vi "ModifyCamGainOnFly.vi"() -> (11 "Waveform Graph":T1(graph)={"Starting Value"=0.0, "Incremental Value"=1.0, "Histogram"=[36, 1982, 49222, 315462, 721902, 687030, 535519, 277999, 136964, 72699, 42936, 24297, 19870, 14020, 10724, 8169, 7364, 6885, 8983, 9078, 8040, 5942, 4163, 2700, 2224, 1518, 1184, 962, 794, 840, 791, 692, 704, 627, 576, 578, 599, 535, 562, 517, 433, 498, 495, 523, 508, 500, 424, 516, 521, 534, 536, 550, 473, 579, 637, 766, 994, 1390, 2263, 3532, 4826, 6338, 7904, 7840, 10087, 11510, 12425, 13291, 14003, 13131, 15643, 16496, 16816, 17351, 17382, 16247, 18117, 19212, 19564, 19906, 20192, 18158, 20845, 21036, 21155, 21500, 19947, 22270, 22427, 22798, 23054, 22885, 21392, 22893, 23378, 22987, 22725, 22279, 20032, 21700, 21318, 21299, 20997, 20581, 17538, 19517, 18720, 18053, 17117, 15803, 13365, 14749, 13814, 12882, 12424, 10652, 11446, 10956, 10453, 10078, 9827, 8214, 9205, 8666, 8580, 8230, 7916, 7053, 7780, 7510, 7481, 7117, 6917, 6085, 6746, 6504, 6528, 6400, 6411, 5847, 6398, 6144, 6240, 6266, 5703, 6278, 6252, 6337, 6214, 6101, 5385, 6384, 6050, 6019, 6049, 6133, 5211, 6033, 5779, 5922, 5892, 5716, 4896, 5698, 5422, 5453, 5196, 5171, 4454, 5128, 4935, 4811, 4703, 4201, 4558, 4619, 4486, 4538, 4519, 3954, 4387, 4328, 4199, 4314, 4236, 3821, 4216, 4202, 4179, 4047, 4159, 3596, 4407, 4327, 4416, 4500, 4534, 3811, 4435, 4379, 4680, 4639, 4093, 4834, 4800, 4889, 5055, 5107, 4555, 5291, 5239, 5274, 5438, 5334, 4579, 5298, 5466, 5556, 5443, 5617, 5245, 5689, 5928, 5903, 6109, 6311, 5731, 6440, 6634, 6784, 6707, 6244, 7026, 7177, 7570, 7403, 7677, 6760, 7926, 7840, 8079, 8447, 8111, 7376, 8176, 8099, 8226, 7974, 7684, 6752, 7643, 7363, 7103, 6900, 6575, 211426]})   [LabVIEW 2016]
uses:
  <vilib>/vision/driver/IMAQdx.llb/IMAQdx Attribute Type.ctl
  <vilib>/vision/driver/IMAQdx.llb/IMAQdx Attribute Visibility.ctl
  <vilib>/vision/driver/NI_Vision_Acquisition_Software.lvlib
  <resource>/objmgr/imaqdx.rc
  <vilib>/vision/NI_Vision_Development_Module.lvlib
panel:
  in  "Gain":dbl(slide)=4.875739644970414 scale=0.0..20.0
  in  "stop":bool
  out "Attribute Information Array":T3(array[cluster])=[{"Attribute Type"=enum."U32", "Readable"=TRUE, "Writable"=TRUE, "Attribute Name"="AcquisitionAttributes::AdvancedGenicam::CommandTimeout"}, {"Attribute Type"=enum."U32", "Readable"=TRUE, "Writable"=TRUE, "Attribute Name"="AcquisitionAttributes::AdvancedGenicam::EventQueueDepth"}, {"Attribute Type"=enum."Bool", "Readable"=TRUE, "Writable"=TRUE, "Attribute Name"="AcquisitionAttributes::AdvancedGenicam::EventsEnabled"}, {"Attribute Type"=enum."Bool", "Readable"=TRUE, "Writable"=FALSE, "Attribute Name"="AcquisitionAttributes::AdvancedGenicam::EventsSupported"}, {"Attribute Type"=enum."Bool", "Readable"=TRUE, "Writable"=TRUE, "Attribute Name"="AcquisitionAttributes::AdvancedGenicam::IgnoreCameraValidationErrors"}, {"Attribute Type"=enum."U32", "Readable"=TRUE, "Writable"=FALSE, "Attribute Name"="AcquisitionAttributes::AdvancedUSB3Vision::ActualMaximumPayloadTransferSize"}, {"Attribute Type"=enum."U32", "Readable"=TRUE, "Writable"=FALSE, "Attribute Name"="AcquisitionAttributes::AdvancedUSB3Vision::RequiredPayloadSizeAlignment"}, {"Attribute Type"=enum."Enum", "Readable"=TRUE, "Writable"=FALSE, "Attribute Name"="AcquisitionAttributes::Bayer::Algorithm"}, {"Attribute Type"=enum."DBL", "Readable"=TRUE, "Writable"=FALSE, "Attribute Name"="AcquisitionAttributes::Bayer::GainB"}, {"Attribute Type"=enum."DBL", "Readable"=TRUE, "Writable"=FALSE, "Attribute Name"="AcquisitionAttributes::Bayer::GainG"}, {"Attribute Type"=enum."DBL", "Readable"=TRUE, "Writable"=FALSE, "Attribute Name"="AcquisitionAttributes::Bayer::GainR"}, {"Attribute Type"=enum."Enum", "Readable"=TRUE, "Writable"=FALSE, "Attribute Name"="AcquisitionAttributes::Bayer::Pattern"}, {"Attribute Type"=enum."Bool", "Readable"=TRUE, "Writable"=FALSE, "Attribute Name"="AcquisitionAttributes::ChunkDataDecoding::ChunkDataDecodingEnabled"}, {"Attribute Type"=enum."U32", "Readable"=TRUE, "Writable"=FALSE, "Attribute Name"="AcquisitionAttributes::ChunkDataDecoding::MaximumChunkCopySize"}, {"Attribute Type"=enum."I64", "Readable"=TRUE, "Writable"=FALSE, "Attribute Name"="CameraAttributes::ImageFormatControl::SensorWidth"}, {"Attribute Type"=enum."I64", "Readable"=TRUE, "Writable"=FALSE, "Attribute Name"="CameraAttributes::ImageFormatControl::SensorHeight"}, {"Attribute Type"=enum."I64", "Readable"=TRUE, "Writable"=FALSE, "Attribute Name"="CameraAttributes::ImageFormatControl::WidthMax"}, {"Attribute Type"=enum."I64", "Readable"=TRUE, "Writable"=FALSE, "Attribute Name"="CameraAttributes::ImageFormatControl::HeightMax"}, {"Attribute Type"=enum."I64", "Readable"=TRUE, "Writable"=FALSE, "Attribute Name"="CameraAttributes::ImageFormatControl::Width"}, {"Attribute Type"=enum."I64", "Readable"=TRUE, "Writable"=FALSE, "Attribute Name"="CameraAttributes::ImageFormatControl::Height"}, {"Attribute Type"=enum."I64", "Readable"=TRUE, "Writable"=TRUE, "Attribute Name"="CameraAttributes::ImageFormatControl::OffsetX"}, {"Attribute Type"=enum."I64", "Readable"=TRUE, "Writable"=TRUE, "Attribute Name"="CameraAttributes::ImageFormatControl::OffsetY"}, {"Attribute Type"=enum."Bool", "Readable"=TRUE, "Writable"=TRUE, "Attribute Name"="CameraAttributes::ImageFormatControl::CenterX"}, {"Attribute Type"=enum."Bool", "Readable"=TRUE, "Writable"=TRUE, "Attribute Name"="CameraAttributes::ImageFormatControl::CenterY"}, {"Attribute Type"=enum."I64", "Readable"=TRUE, "Writable"=FALSE, "Attribute Name"="CameraAttributes::ImageFormatControl::BinningHorizontal"}, {"Attribute Type"=enum."I64", "Readable"=TRUE, "Writable"=FALSE, "Attribute Name"="CameraAttributes::ImageFormatControl::BinningVertical"}, {"Attribute Type"=enum."Bool", "Readable"=TRUE, "Writable"=TRUE, "Attribute Name"="CameraAttributes::ImageFormatControl::ReverseX"}, {"Attribute Type"=enum."Enum", "Readable"=TRUE, "Writable"=FALSE, "Attribute Name"="CameraAttributes::ImageFormatControl::PixelFormat"}, {"Attribute Type"=enum."Enum", "Readable"=TRUE, "Writable"=FALSE, "Attribute Name"="CameraAttributes::ImageFormatControl::PixelSize"}, {"Attribute Type"=enum."Enum", "Readable"=TRUE, "Writable"=FALSE, "Attribute Name"="CameraAttributes::ImageFormatControl::PixelColorFilter"}, {"Attribute Type"=enum."I64", "Readable"=TRUE, "Writable"=FALSE, "Attribute Name"="CameraAttributes::ImageFormatControl::PixelDynamicRangeMin"}, {"Attribute Type"=enum."I64", "Readable"=TRUE, "Writable"=FALSE, "Attribute Name"="CameraAttributes::ImageFormatControl::PixelDynamicRangeMax"}, {"Attribute Type"=enum."Enum", "Readable"=TRUE, "Writable"=TRUE, "Attribute Name"="CameraAttributes::ImageFormatControl::TestImageSelector"}, {"Attribute Type"=enum."Enum", "Readable"=TRUE, "Writable"=TRUE, "Attribute Name"="CameraAttributes::AnalogControl::GainAuto"}, {"Attribute Type"=enum."Enum", "Readable"=TRUE, "Writable"=TRUE, "Attribute Name"="CameraAttributes::AnalogControl::GainSelector"}, {"Attribute Type"=enum."DBL", "Readable"=TRUE, "Writable"=TRUE, "Attribute Name"="CameraAttributes::AnalogControl::Gain"}, {"Attribute Type"=enum."Enum", "Readable"=TRUE, "Writable"=TRUE, "Attribute Name"="CameraAttributes::AnalogControl::BlackLevelSelector"}, {"Attribute Type"=enum."DBL", "Readable"=TRUE, "Writable"=TRUE, "Attribute Name"="CameraAttributes::AnalogControl::BlackLevel"}, {"Attribute Type"=enum."DBL", "Readable"=TRUE, "Writable"=TRUE, "Attribute Name"="CameraAttributes::AnalogControl::Gamma"}, {"Attribute Type"=enum."I64", "Readable"=TRUE, "Writable"=TRUE, "Attribute Name"="CameraAttributes::AnalogControl::DigitalShift"}, {"Attribute Type"=enum."DBL", "Readable"=FALSE, "Writable"=FALSE, "Attribute Name"="CameraAttributes::ImageQualityControl::ColorTransformationValue"}, {"Attribute Type"=enum."Enum", "Readable"=TRUE, "Writable"=FALSE, "Attribute Name"="CameraAttributes::AcquisitionControl::AcquisitionMode"}, {"Attribute Type"=enum."Enum", "Readable"=TRUE, "Writable"=TRUE, "Attribute Name"="CameraAttributes::AcquisitionControl::ShutterMode"}, {"Attribute Type"=enum."Enum", "Readable"=TRUE, "Writable"=TRUE, "Attribute Name"="CameraAttributes::AcquisitionControl::ExposureAuto"}, {"Attribute Type"=enum."Enum", "Readable"=TRUE, "Writable"=TRUE, "Attribute Name"="CameraAttributes::AcquisitionControl::ExposureMode"}, {"Attribute Type"=enum."DBL", "Readable"=TRUE, "Writable"=TRUE, "Attribute Name"="CameraAttributes::AcquisitionControl::ExposureTime"}, {"Attribute Type"=enum."I64", "Readable"=TRUE, "Writable"=FALSE, "Attribute Name"="CameraAttributes::AcquisitionControl::AcquisitionBurstFrameCount"}, {"Attribute Type"=enum."Enum", "Readable"=TRUE, "Writable"=TRUE, "Attribute Name"="CameraAttributes::AcquisitionControl::TriggerSelector"}, {"Attribute Type"=enum."Enum", "Readable"=TRUE, "Writable"=TRUE, "Attribute Name"="CameraAttributes::AcquisitionControl::TriggerMode"}, {"Attribute Type"=enum."Command", "Readable"=FALSE, "Writable"=TRUE, "Attribute Name"="CameraAttributes::AcquisitionControl::TriggerSoftware"}, {"Attribute Type"=enum."Enum", "Readable"=TRUE, "Writable"=TRUE, "Attribute Name"="CameraAttributes::AcquisitionControl::TriggerSource"}, {"Attribute Type"=enum."Enum", "Readable"=TRUE, "Writable"=TRUE, "Attribute Name"="CameraAttributes::AcquisitionControl::TriggerActivation"}, {"Attribute Type"=enum."DBL", "Readable"=TRUE, "Writable"=TRUE, "Attribute Name"="CameraAttributes::AcquisitionControl::TriggerDelay"}, {"Attribute Type"=enum."Bool", "Readable"=TRUE, "Writable"=TRUE, "Attribute Name"="CameraAttributes::AcquisitionControl::AcquisitionFrameRateEnable"}, {"Attribute Type"=enum."DBL", "Readable"=TRUE, "Writable"=TRUE, "Attribute Name"="CameraAttributes::AcquisitionControl::AcquisitionFrameRate"}, {"Attribute Type"=enum."DBL", "Readable"=TRUE, "Writable"=FALSE, "Attribute Name"="CameraAttributes::AcquisitionControl::ResultingFrameRate"}, {"Attribute Type"=enum."DBL", "Readable"=TRUE, "Writable"=FALSE, "Attribute Name"="CameraAttributes::AcquisitionControl::SensorReadoutTime"}, {"Attribute Type"=enum."Enum", "Readable"=TRUE, "Writable"=TRUE, "Attribute Name"="CameraAttributes::AcquisitionControl::AcquisitionStatusSelector"}, {"Attribute Type"=enum."Bool", "Readable"=TRUE, "Writable"=FALSE, "Attribute Name"="CameraAttributes::AcquisitionControl::AcquisitionStatus"}, {"Attribute Type"=enum."DBL", "Readable"=TRUE, "Writable"=TRUE, "Attribute Name"="CameraAttributes::AutoFunctionControl::AutoTargetBrightness"}, {"Attribute Type"=enum."Enum", "Readable"=TRUE, "Writable"=TRUE, "Attribute Name"="CameraAttributes::AutoFunctionControl::AutoFunctionProfile"}, {"Attribute Type"=enum."DBL", "Readable"=TRUE, "Writable"=TRUE, "Attribute Name"="CameraAttributes::AutoFunctionControl::AutoGainLowerLimit"}, {"Attribute Type"=enum."DBL", "Readable"=TRUE, "Writable"=TRUE, "Attribute Name"="CameraAttributes::AutoFunctionControl::AutoGainUpperLimit"}, {"Attribute Type"=enum."DBL", "Readable"=TRUE, "Writable"=TRUE, "Attribute Name"="CameraAttributes::AutoFunctionControl::AutoExposureTimeLowerLimit"}, {"Attribute Type"=enum."DBL", "Readable"=TRUE, "Writable"=TRUE, "Attribute Name"="CameraAttributes::AutoFunctionControl::AutoExposureTimeUpperLimit"}, {"Attribute Type"=enum."Enum", "Readable"=TRUE, "Writable"=TRUE, "Attribute Name"="CameraAttributes::AutoFunctionControl::AutoFunctionAOIControl::AutoFunctionAOISelector"}, {"Attribute Type"=enum."I64", "Readable"=TRUE, "Writable"=TRUE, "Attribute Name"="CameraAttributes::AutoFunctionControl::AutoFunctionAOIControl::AutoFunctionAOIWidth"}, {"Attribute Type"=enum."I64", "Readable"=TRUE, "Writable"=TRUE, "Attribute Name"="CameraAttributes::AutoFunctionControl::AutoFunctionAOIControl::AutoFunctionAOIHeight"}, {"Attribute Type"=enum."I64", "Readable"=TRUE, "Writable"=TRUE, "Attribute Name"="CameraAttributes::AutoFunctionControl::AutoFunctionAOIControl::AutoFunctionAOIOffsetX"}, {"Attribute Type"=enum."I64", "Readable"=TRUE, "Writable"=TRUE, "Attribute Name"="CameraAttributes::AutoFunctionControl::AutoFunctionAOIControl::AutoFunctionAOIOffsetY"}, {"Attribute Type"=enum."Bool", "Readable"=TRUE, "Writable"=TRUE, "Attribute Name"="CameraAttributes::AutoFunctionControl::AutoFunctionAOIControl::AutoFunctionAOIUseBrightness"}, {"Attribute Type"=enum."Bool", "Readable"=TRUE, "Writable"=TRUE, "Attribute Name"="CameraAttributes::AutoFunctionControl::AutoFunctionAOIControl::AutoFunctionAOIUseWhiteBalance"}, {"Attribute Type"=enum."Enum", "Readable"=TRUE, "Writable"=TRUE, "Attribute Name"="CameraAttributes::LUTControl::LUTSelector"}, {"Attribute Type"=enum."Bool", "Readable"=TRUE, "Writable"=TRUE, "Attribute Name"="CameraAttributes::LUTControl::LUTEnable"}, {"Attribute Type"=enum."I64", "Readable"=TRUE, "Writable"=TRUE, "Attribute Name"="CameraAttributes::LUTControl::LUTIndex"}, {"Attribute Type"=enum."I64", "Readable"=TRUE, "Writable"=TRUE, "Attribute Name"="CameraAttributes::LUTControl::LUTValue"}, {"Attribute Type"=enum."Enum", "Readable"=TRUE, "Writable"=TRUE, "Attribute Name"="CameraAttributes::DigitalIOControl::LineSelector"}, {"Attribute Type"=enum."Enum", "Readable"=TRUE, "Writable"=TRUE, "Attribute Name"="CameraAttributes::DigitalIOControl::LineMode"}, {"Attribute Type"=enum."Enum", "Readable"=TRUE, "Writable"=FALSE, "Attribute Name"="CameraAttributes::DigitalIOControl::LineFormat"}, {"Attribute Type"=enum."Enum", "Readable"=TRUE, "Writable"=FALSE, "Attribute Name"="CameraAttributes::DigitalIOControl::LineLogic"}, {"Attribute Type"=enum."Enum", "Readable"=FALSE, "Writable"=FALSE, "Attribute Name"="CameraAttributes::DigitalIOControl::LineSource"}, {"Attribute Type"=enum."Bool", "Readable"=TRUE, "Writable"=TRUE, "Attribute Name"="CameraAttributes::DigitalIOControl::LineInverter"}, {"Attribute Type"=enum."DBL", "Readable"=TRUE, "Writable"=TRUE, "Attribute Name"="CameraAttributes::DigitalIOControl::LineDebouncerTime"}, {"Attribute Type"=enum."DBL", "Readable"=FALSE, "Writable"=FALSE, "Attribute Name"="CameraAttributes::DigitalIOControl::LineMinimumOutputPulseWidth"}, {"Attribute Type"=enum."Bool", "Readable"=FALSE, "Writable"=FALSE, "Attribute Name"="CameraAttributes::DigitalIOControl::LineOverloadStatus"}, {"Attribute Type"=enum."Bool", "Readable"=TRUE, "Writable"=FALSE, "Attribute Name"="CameraAttributes::DigitalIOControl::LineStatus"}, {"Attribute Type"=enum."I64", "Readable"=TRUE, "Writable"=FALSE, "Attribute Name"="CameraAttributes::DigitalIOControl::LineStatusAll"}, {"Attribute Type"=enum."Enum", "Readable"=TRUE, "Writable"=TRUE, "Attribute Name"="CameraAttributes::DigitalIOControl::UserOutputSelector"}, {"Attribute Type"=enum."Bool", "Readable"=TRUE, "Writable"=TRUE, "Attribute Name"="CameraAttributes::DigitalIOControl::UserOutputValue"}, {"Attribute Type"=enum."I64", "Readable"=TRUE, "Writable"=TRUE, "Attribute Name"="CameraAttributes::DigitalIOControl::UserOutputValueAll"}, {"Attribute Type"=enum."Enum", "Readable"=TRUE, "Writable"=TRUE, "Attribute Name"="CameraAttributes::CounterAndTimerControl::TimerSelector"}, {"Attribute Type"=enum."DBL", "Readable"=TRUE, "Writable"=TRUE, "Attribute Name"="CameraAttributes::CounterAndTimerControl::TimerDuration"}, {"Attribute Type"=enum."DBL", "Readable"=TRUE, "Writable"=TRUE, "Attribute Name"="CameraAttributes::CounterAndTimerControl::TimerDelay"}, {"Attribute Type"=enum."Enum", "Readable"=TRUE, "Writable"=TRUE, "Attribute Name"="CameraAttributes::CounterAndTimerControl::TimerTriggerSource"}, {"Attribute Type"=enum."Enum", "Readable"=TRUE, "Writable"=TRUE, "Attribute Name"="CameraAttributes::CounterAndTimerControl::CounterSelector"}, {"Attribute Type"=enum."Enum", "Readable"=TRUE, "Writable"=TRUE, "Attribute Name"="CameraAttributes::CounterAndTimerControl::CounterEventSource"}, {"Attribute Type"=enum."Enum", "Readable"=TRUE, "Writable"=TRUE, "Attribute Name"="CameraAttributes::CounterAndTimerControl::CounterResetSource"}, {"Attribute Type"=enum."Enum", "Readable"=TRUE, "Writable"=TRUE, "Attribute Name"="CameraAttributes::CounterAndTimerControl::CounterResetActivation"}, {"Attribute Type"=enum."Command", "Readable"=FALSE, "Writable"=FALSE, "Attribute Name"="CameraAttributes::CounterAndTimerControl::CounterReset"}, {"Attribute Type"=enum."Bool", "Readable"=TRUE, "Writable"=FALSE, "Attribute Name"="CameraAttributes::ChunkDataControl::ChunkModeActive"}, {"Attribute Type"=enum."Enum", "Readable"=TRUE, "Writable"=TRUE, "Attribute Name"="CameraAttributes::ChunkDataControl::ChunkSelector"}, {"Attribute Type"=enum."Bool", "Readable"=TRUE, "Writable"=FALSE, "Attribute Name"="CameraAttributes::ChunkDataControl::ChunkEnable"}, {"Attribute Type"=enum."Enum", "Readable"=FALSE, "Writable"=FALSE, "Attribute Name"="CameraAttributes::ChunkDataControl::ChunkGainSelector"}, {"Attribute Type"=enum."DBL", "Readable"=FALSE, "Writable"=FALSE, "Attribute Name"="CameraAttributes::ChunkDataControl::ChunkGain"}, {"Attribute Type"=enum."DBL", "Readable"=FALSE, "Writable"=FALSE, "Attribute Name"="CameraAttributes::ChunkDataControl::ChunkExposureTime"}, {"Attribute Type"=enum."I64", "Readable"=FALSE, "Writable"=FALSE, "Attribute Name"="CameraAttributes::ChunkDataControl::ChunkTimestamp"}, {"Attribute Type"=enum."I64", "Readable"=FALSE, "Writable"=FALSE, "Attribute Name"="CameraAttributes::ChunkDataControl::ChunkPayloadCRC16"}, {"Attribute Type"=enum."Enum", "Readable"=FALSE, "Writable"=FALSE, "Attribute Name"="CameraAttributes::ChunkDataControl::ChunkCounterSelector"}, {"Attribute Type"=enum."I64", "Readable"=FALSE, "Writable"=FALSE, "Attribute Name"="CameraAttributes::ChunkDataControl::ChunkCounterValue"}, {"Attribute Type"=enum."Enum", "Readable"=FALSE, "Writable"=FALSE, "Attribute Name"="CameraAttributes::ChunkDataControl::ChunkData::ChunkGainSelector"}, {"Attribute Type"=enum."DBL", "Readable"=FALSE, "Writable"=FALSE, "Attribute Name"="CameraAttributes::ChunkDataControl::ChunkData::ChunkGain"}, {"Attribute Type"=enum."DBL", "Readable"=FALSE, "Writable"=FALSE, "Attribute Name"="CameraAttributes::ChunkDataControl::ChunkData::ChunkExposureTime"}, {"Attribute Type"=enum."I64", "Readable"=FALSE, "Writable"=FALSE, "Attribute Name"="CameraAttributes::ChunkDataControl::ChunkData::ChunkTimestamp"}, {"Attribute Type"=enum."I64", "Readable"=FALSE, "Writable"=FALSE, "Attribute Name"="CameraAttributes::ChunkDataControl::ChunkData::ChunkPayloadCRC16"}, {"Attribute Type"=enum."Enum", "Readable"=FALSE, "Writable"=FALSE, "Attribute Name"="CameraAttributes::ChunkDataControl::ChunkData::ChunkCounterSelector"}, {"Attribute Type"=enum."I64", "Readable"=FALSE, "Writable"=FALSE, "Attribute Name"="CameraAttributes::ChunkDataControl::ChunkData::ChunkCounterValue"}, {"Attribute Type"=enum."Enum", "Readable"=TRUE, "Writable"=TRUE, "Attribute Name"="CameraAttributes::EventControl::EventSelector"}, {"Attribute Type"=enum."Enum", "Readable"=TRUE, "Writable"=TRUE, "Attribute Name"="CameraAttributes::EventControl::EventNotification"}, {"Attribute Type"=enum."I64", "Readable"=FALSE, "Writable"=FALSE, "Attribute Name"="CameraAttributes::EventControl::EventExposureEndData::EventExposureEnd"}, {"Attribute Type"=enum."I64", "Readable"=FALSE, "Writable"=FALSE, "Attribute Name"="CameraAttributes::EventControl::EventExposureEndData::EventExposureEndTimestamp"}, {"Attribute Type"=enum."I64", "Readable"=FALSE, "Writable"=FALSE, "Attribute Name"="CameraAttributes::EventControl::EventExposureEndData::EventExposureEndFrameID"}, {"Attribute Type"=enum."I64", "Readable"=FALSE, "Writable"=FALSE, "Attribute Name"="CameraAttributes::EventControl::EventFrameStartData::EventFrameStart"}, {"Attribute Type"=enum."I64", "Readable"=FALSE, "Writable"=FALSE, "Attribute Name"="CameraAttributes::EventControl::EventFrameStartData::EventFrameStartTimestamp"}, {"Attribute Type"=enum."I64", "Readable"=FALSE, "Writable"=FALSE, "Attribute Name"="CameraAttributes::EventControl::EventFrameStartData::EventFrameStartFrameID"}, {"Attribute Type"=enum."I64", "Readable"=FALSE, "Writable"=FALSE, "Attribute Name"="CameraAttributes::EventControl::EventFrameBurstStartData::EventFrameBurstStart"}, {"Attribute Type"=enum."I64", "Readable"=FALSE, "Writable"=FALSE, "Attribute Name"="CameraAttributes::EventControl::EventFrameBurstStartData::EventFrameBurstStartTimestamp"}, {"Attribute Type"=enum."I64", "Readable"=FALSE, "Writable"=FALSE, "Attribute Name"="CameraAttributes::EventControl::EventFrameBurstStartData::EventFrameBurstStartFrameID"}, {"Attribute Type"=enum."I64", "Readable"=FALSE, "Writable"=FALSE, "Attribute Name"="CameraAttributes::EventControl::EventFrameStartOvertriggerData::EventFrameStartOvertrigger"}, {"Attribute Type"=enum."I64", "Readable"=FALSE, "Writable"=FALSE, "Attribute Name"="CameraAttributes::EventControl::EventFrameStartOvertriggerData::EventFrameStartOvertriggerTimestamp"}, {"Attribute Type"=enum."I64", "Readable"=FALSE, "Writable"=FALSE, "Attribute Name"="CameraAttributes::EventControl::EventFrameStartOvertriggerData::EventFrameStartOvertriggerFrameID"}, {"Attribute Type"=enum."I64", "Readable"=FALSE, "Writable"=FALSE, "Attribute Name"="CameraAttributes::EventControl::EventFrameBurstStartOvertriggerData::EventFrameBurstStartOvertrigger"}, {"Attribute Type"=enum."I64", "Readable"=FALSE, "Writable"=FALSE, "Attribute Name"="CameraAttributes::EventControl::EventFrameBurstStartOvertriggerData::EventFrameBurstStartOvertriggerTimestamp"}, {"Attribute Type"=enum."I64", "Readable"=FALSE, "Writable"=FALSE, "Attribute Name"="CameraAttributes::EventControl::EventFrameBurstStartOvertriggerData::EventFrameBurstStartOvertriggerFrameID"}, {"Attribute Type"=enum."Enum", "Readable"=TRUE, "Writable"=FALSE, "Attribute Name"="CameraAttributes::UserSetControl::UserSetSelector"}, {"Attribute Type"=enum."Command", "Readable"=FALSE, "Writable"=TRUE, "Attribute Name"="CameraAttributes::UserSetControl::UserSetLoad"}, {"Attribute Type"=enum."Command", "Readable"=FALSE, "Writable"=TRUE, "Attribute Name"="CameraAttributes::UserSetControl::UserSetSave"}, {"Attribute Type"=enum."Enum", "Readable"=TRUE, "Writable"=FALSE, "Attribute Name"="CameraAttributes::UserSetControl::UserSetDefault"}, {"Attribute Type"=enum."I64", "Readable"=TRUE, "Writable"=FALSE, "Attribute Name"="CameraAttributes::TransportLayerControl::PayloadSize"}, {"Attribute Type"=enum."Enum", "Readable"=TRUE, "Writable"=FALSE, "Attribute Name"="CameraAttributes::TransportLayerControl::BslUSBSpeedMode"}, {"Attribute Type"=enum."I64", "Readable"=TRUE, "Writable"=FALSE, "Attribute Name"="CameraAttributes::TransportLayerControl::SIPayloadTransferSize"}, {"Attribute Type"=enum."I64", "Readable"=TRUE, "Writable"=FALSE, "Attribute Name"="CameraAttributes::TransportLayerControl::SIPayloadTransferCount"}, {"Attribute Type"=enum."I64", "Readable"=TRUE, "Writable"=FALSE, "Attribute Name"="CameraAttributes::TransportLayerControl::SIPayloadFinalTransfer1Size"}, {"Attribute Type"=enum."I64", "Readable"=TRUE, "Writable"=FALSE, "Attribute Name"="CameraAttributes::TransportLayerControl::SIPayloadFinalTransfer2Size"}, {"Attribute Type"=enum."String", "Readable"=TRUE, "Writable"=FALSE, "Attribute Name"="CameraAttributes::DeviceControl::DeviceVendorName"}, {"Attribute Type"=enum."String", "Readable"=TRUE, "Writable"=FALSE, "Attribute Name"="CameraAttributes::DeviceControl::DeviceModelName"}, {"Attribute Type"=enum."String", "Readable"=TRUE, "Writable"=FALSE, "Attribute Name"="CameraAttributes::DeviceControl::DeviceManufacturerInfo"}, {"Attribute Type"=enum."String", "Readable"=TRUE, "Writable"=FALSE, "Attribute Name"="CameraAttributes::DeviceControl::DeviceVersion"}, {"Attribute Type"=enum."String", "Readable"=TRUE, "Writable"=FALSE, "Attribute Name"="CameraAttributes::DeviceControl::DeviceFirmwareVersion"}, {"Attribute Type"=enum."String", "Readable"=TRUE, "Writable"=FALSE, "Attribute Name"="CameraAttributes::DeviceControl::DeviceSerialNumber"}, {"Attribute Type"=enum."String", "Readable"=TRUE, "Writable"=TRUE, "Attribute Name"="CameraAttributes::DeviceControl::DeviceUserID"}, {"Attribute Type"=enum."Enum", "Readable"=TRUE, "Writable"=FALSE, "Attribute Name"="CameraAttributes::DeviceControl::DeviceScanType"}, {"Attribute Type"=enum."I64", "Readable"=TRUE, "Writable"=TRUE, "Attribute Name"="CameraAttributes::DeviceControl::DeviceLinkSelector"}, {"Attribute Type"=enum."I64", "Readable"=TRUE, "Writable"=FALSE, "Attribute Name"="CameraAttributes::DeviceControl::DeviceLinkSpeed"}, {"Attribute Type"=enum."Enum", "Readable"=TRUE, "Writable"=TRUE, "Attribute Name"="CameraAttributes::DeviceControl::DeviceLinkThroughputLimitMode"}, {"Attribute Type"=enum."I64", "Readable"=TRUE, "Writable"=TRUE, "Attribute Name"="CameraAttributes::DeviceControl::DeviceLinkThroughputLimit"}, {"Attribute Type"=enum."I64", "Readable"=TRUE, "Writable"=FALSE, "Attribute Name"="CameraAttributes::DeviceControl::DeviceLinkCurrentThroughput"}, {"Attribute Type"=enum."I64", "Readable"=TRUE, "Writable"=FALSE, "Attribute Name"="CameraAttributes::DeviceControl::DeviceSFNCVersionMajor"}, {"Attribute Type"=enum."I64", "Readable"=TRUE, "Writable"=FALSE, "Attribute Name"="CameraAttributes::DeviceControl::DeviceSFNCVersionMinor"}, {"Attribute Type"=enum."I64", "Readable"=TRUE, "Writable"=FALSE, "Attribute Name"="CameraAttributes::DeviceControl::DeviceSFNCVersionSubMinor"}, {"Attribute Type"=enum."Enum", "Readable"=TRUE, "Writable"=TRUE, "Attribute Name"="CameraAttributes::UserDefinedValueControl::UserDefinedValueSelector"}, {"Attribute Type"=enum."I64", "Readable"=TRUE, "Writable"=TRUE, "Attribute Name"="CameraAttributes::UserDefinedValueControl::UserDefinedValue"}, {"Attribute Type"=enum."Enum", "Readable"=TRUE, "Writable"=TRUE, "Attribute Name"="CameraAttributes::RemoveParameterLimitControl::RemoveParameterLimitSelector"}, {"Attribute Type"=enum."Bool", "Readable"=TRUE, "Writable"=TRUE, "Attribute Name"="CameraAttributes::RemoveParameterLimitControl::RemoveParameterLimit"}, {"Attribute Type"=enum."Enum", "Readable"=TRUE, "Writable"=TRUE, "Attribute Name"="CameraAttributes::ExpertFeatureAccess::ExpertFeatureAccessSelector"}, {"Attribute Type"=enum."I64", "Readable"=TRUE, "Writable"=TRUE, "Attribute Name"="CameraAttributes::ExpertFeatureAccess::ExpertFeatureAccessKey"}, {"Attribute Type"=enum."Bool", "Readable"=FALSE, "Writable"=FALSE, "Attribute Name"="CameraAttributes::ExpertFeatureAccess::ExpertFeatureEnable"}, {"Attribute Type"=enum."Enum", "Readable"=TRUE, "Writable"=TRUE, "Attribute Name"="CameraAttributes::FileAccessControl::FileSelector"}, {"Attribute Type"=enum."Enum", "Readable"=TRUE, "Writable"=TRUE, "Attribute Name"="CameraAttributes::FileAccessControl::FileOperationSelector"}, {"Attribute Type"=enum."Enum", "Readable"=TRUE, "Writable"=TRUE, "Attribute Name"="CameraAttributes::FileAccessControl::FileOpenMode"}, {"Attribute Type"=enum."I64", "Readable"=TRUE, "Writable"=TRUE, "Attribute Name"="CameraAttributes::FileAccessControl::FileAccessOffset"}, {"Attribute Type"=enum."I64", "Readable"=TRUE, "Writable"=TRUE, "Attribute Name"="CameraAttributes::FileAccessControl::FileAccessLength"}, {"Attribute Type"=enum."Enum", "Readable"=TRUE, "Writable"=FALSE, "Attribute Name"="CameraAttributes::FileAccessControl::FileOperationStatus"}, {"Attribute Type"=enum."I64", "Readable"=TRUE, "Writable"=FALSE, "Attribute Name"="CameraAttributes::FileAccessControl::FileOperationResult"}, {"Attribute Type"=enum."I64", "Readable"=TRUE, "Writable"=FALSE, "Attribute Name"="CameraAttributes::FileAccessControl::FileSize"}, {"Attribute Type"=enum."Command", "Readable"=FALSE, "Writable"=TRUE, "Attribute Name"="CameraAttributes::FileAccessControl::FileOperationExecute"}, {"Attribute Type"=enum."Enum", "Readable"=TRUE, "Writable"=FALSE, "Attribute Name"="AcquisitionAttributes::BitsPerPixel"}, {"Attribute Type"=enum."Enum", "Readable"=TRUE, "Writable"=FALSE, "Attribute Name"="AcquisitionAttributes::ImageDecoderCopyMode"}, {"Attribute Type"=enum."Enum", "Readable"=TRUE, "Writable"=FALSE, "Attribute Name"="AcquisitionAttributes::IncompleteBufferMode"}, {"Attribute Type"=enum."Enum", "Readable"=TRUE, "Writable"=FALSE, "Attribute Name"="AcquisitionAttributes::OutputImageType"}, {"Attribute Type"=enum."Enum", "Readable"=TRUE, "Writable"=FALSE, "Attribute Name"="AcquisitionAttributes::OverwriteMode"}, {"Attribute Type"=enum."Enum", "Readable"=TRUE, "Writable"=FALSE, "Attribute Name"="AcquisitionAttributes::ReceiveTimestampMode"}, {"Attribute Type"=enum."Bool", "Readable"=TRUE, "Writable"=FALSE, "Attribute Name"="AcquisitionAttributes::ShiftPixelBits"}, {"Attribute Type"=enum."Bool", "Readable"=TRUE, "Writable"=FALSE, "Attribute Name"="AcquisitionAttributes::SwapPixelBytes"}, {"Attribute Type"=enum."U32", "Readable"=TRUE, "Writable"=FALSE, "Attribute Name"="AcquisitionAttributes::Timeout"}, {"Attribute Type"=enum."U32", "Readable"=TRUE, "Writable"=FALSE, "Attribute Name"="CameraInformation::BaseAddress"}, {"Attribute Type"=enum."Enum", "Readable"=TRUE, "Writable"=FALSE, "Attribute Name"="CameraInformation::BusType"}, {"Attribute Type"=enum."String", "Readable"=TRUE, "Writable"=FALSE, "Attribute Name"="CameraInformation::ModelName"}, {"Attribute Type"=enum."String", "Readable"=TRUE, "Writable"=FALSE, "Attribute Name"="CameraInformation::PrimaryURLString"}, {"Attribute Type"=enum."String", "Readable"=TRUE, "Writable"=FALSE, "Attribute Name"="CameraInformation::SecondaryURLString"}, {"Attribute Type"=enum."U32", "Readable"=TRUE, "Writable"=FALSE, "Attribute Name"="CameraInformation::SerialNumberHigh"}, {"Attribute Type"=enum."U32", "Readable"=TRUE, "Writable"=FALSE, "Attribute Name"="CameraInformation::SerialNumberLow"}, {"Attribute Type"=enum."Enum", "Readable"=TRUE, "Writable"=FALSE, "Attribute Name"="CameraInformation::USBConnectionSpeed"}, {"Attribute Type"=enum."String", "Readable"=TRUE, "Writable"=FALSE, "Attribute Name"="CameraInformation::VendorName"}, {"Attribute Type"=enum."Bool", "Readable"=TRUE, "Writable"=FALSE, "Attribute Name"="StatusInformation::AcqInProgress"}, {"Attribute Type"=enum."I64", "Readable"=TRUE, "Writable"=FALSE, "Attribute Name"="StatusInformation::HandledEventCount"}, {"Attribute Type"=enum."I64", "Readable"=TRUE, "Writable"=FALSE, "Attribute Name"="StatusInformation::IncompleteBufferCount"}, {"Attribute Type"=enum."I64", "Readable"=TRUE, "Writable"=FALSE, "Attribute Name"="StatusInformation::LastBufferCount"}, {"Attribute Type"=enum."U32", "Readable"=TRUE, "Writable"=FALSE, "Attribute Name"="StatusInformation::LastBufferNumber"}, {"Attribute Type"=enum."I64", "Readable"=TRUE, "Writable"=FALSE, "Attribute Name"="StatusInformation::LostBufferCount"}, {"Attribute Type"=enum."I64", "Readable"=TRUE, "Writable"=FALSE, "Attribute Name"="StatusInformation::LostEventCount"}]
  out "Image Out":T4(plugin-control)
  in  "Camera Name":refnum<k21>="cam0" caption="IMAQdx Session"
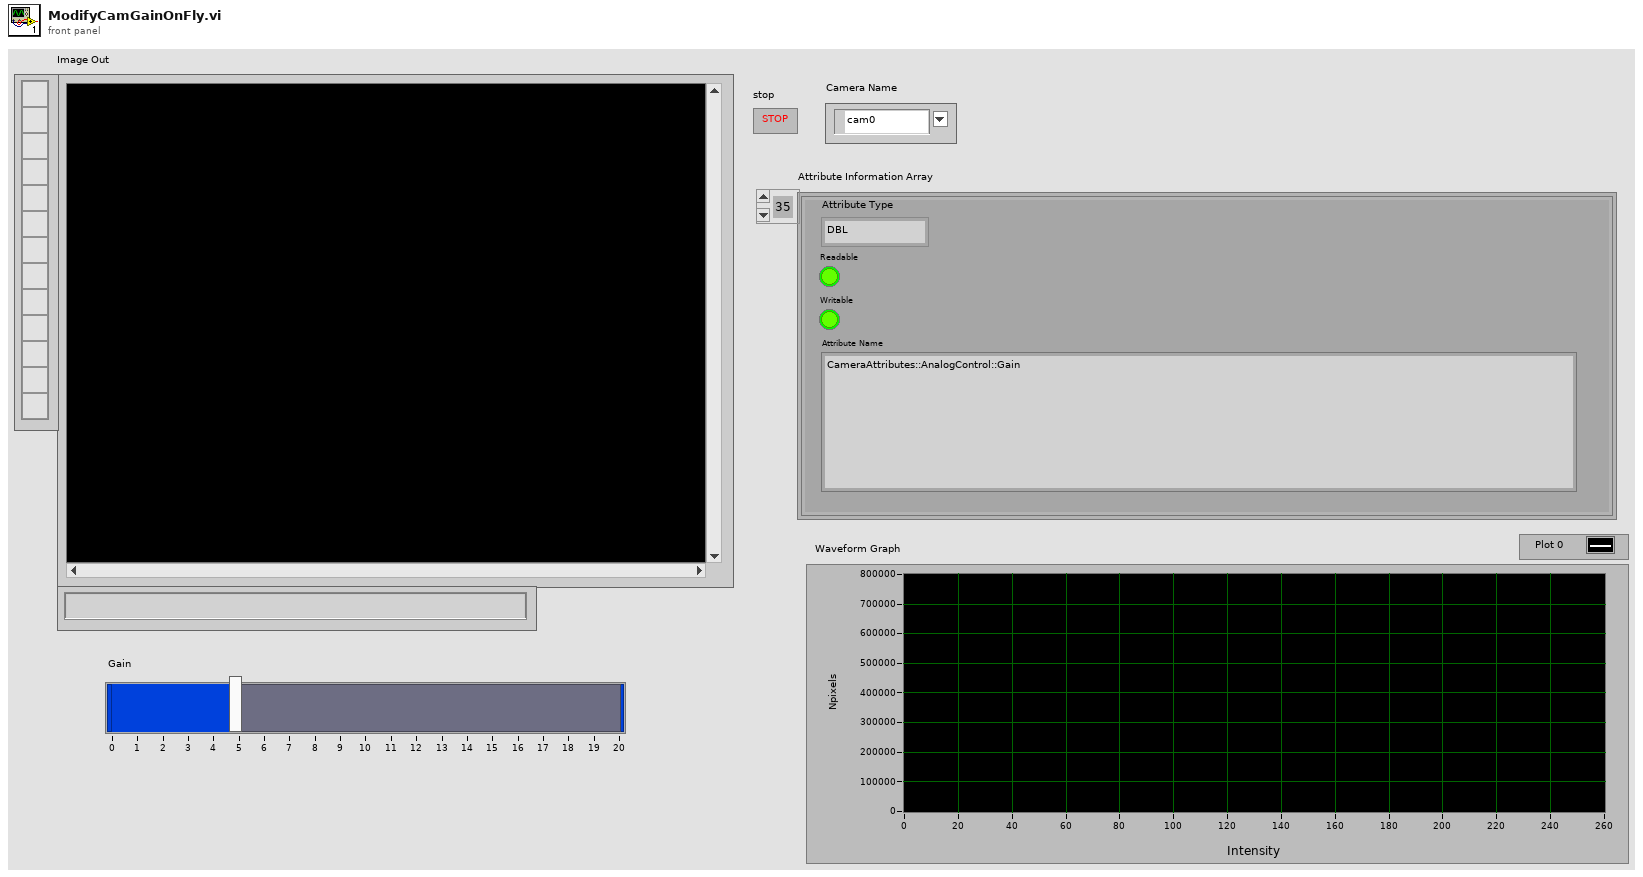
[diagram p1: front panel]
types:
  T1 = cluster{"Starting Value":sgl, "Incremental Value":sgl, "Histogram":u32[]}
  T2 = typedef "NI_Vision_Acquisition_Software.lvlib/IMAQdx Attribute Type.ctl" = enum32{"U32", "I64", "DBL", "String", "Enum", "Bool", "Command"}
  T3 = cluster{"Attribute Type":T2, "Readable":bool, "Writable":bool, "Attribute Name":string}[]
  T4 = typedef "IMAQ Image.ctl" = refnum<image>
  T5 = typedef "Image Type" = u32
  T6 = typedef "IMAQdx.ctl" = refnum<k21>
  T7 = typedef "NI_Vision_Acquisition_Software.lvlib/IMAQdx Attribute Visibility.ctl" = enum32{"Simple", "Intermediate", "Advanced"}
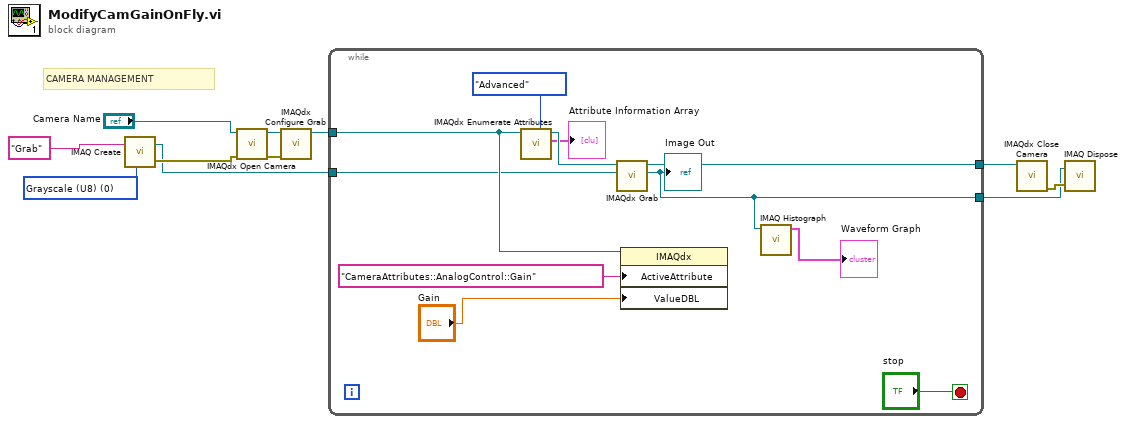
[diagram p0: block diagram]
diagram:
  w6 = T5 0 items=["Grayscale (U8)", "Grayscale (I16)", "Grayscale (SGL)", "Complex (CSG)", "RGB (U32)", "HSL (U32)", "RGB (U64)", "Grayscale (U16)"] ("Image Type")
  # "CAMERA MANAGEMENT"
  n1 = call "IMAQ Create"("Image Name"="Grab", "Image Type"=w6) -> ("New Image"=w4:T4, "error out"=w11:errorcluster)  [unwired: 2 in, 1 out]
  n2 = call <vilib>:"IMAQdx Open Camera.vi"("error in"=w11, "Session In"="Camera Name") -> ("error out"=w8:errorcluster, "Session Out"=w9:T6)  [unwired: 1 in, 7 out]
  n3 = call <vilib>:"IMAQdx Configure Grab.vi"("error in"=w8, "Session In"=w9) -> ("Session Out"=w5:T6)  [unwired: 9 out]
  n4 = while {
    tunnel: w5 -> [w22]
    tunnel: w4 -> [w20]
    tunnel: [w17] -> w3
    tunnel: [w13] -> w1
    stop <- "stop" stop-if-true
    n5 = call <vilib>:"IMAQdx Enumerate Attributes.vi"("Visibility"=IMAQdx_Attribute_Visibility."Advanced", "Session In"=w22) -> ("Attribute Information Array"=→"Attribute Information Array":T3, "Session Out"=w21:T6)  [unwired: 7 in, 1 out]
    n6 = call <vilib>:"IMAQdx Grab.vi"("Image In"=w20, "Session In"=w21) -> ("Image Out"=w13:T4, "Session Out"=w17:T6)  [unwired: 2 in, 6 out]
    "Image Out" <- w13
    n7 = property class="IMAQdx"(reference=w22, "ActiveAttribute"="CameraAttributes::AnalogControl::Gain", "ValueDBL"="Gain") -> ()  [unwired: 1 in, 2 out]
    n8 = call "IMAQ Histograph"("Image"=w13) -> ("Histogram Graph"=→"Waveform Graph":T1)  [unwired: 7 in, 3 out]
  }
  n9 = call <vilib>:"IMAQdx Close Camera.vi"("Session In"=w3) -> ("error out"=w2:errorcluster)  [unwired: 10 in]
  n10 = call "IMAQ Dispose"("Image"=w1, "error in (no error)"=w2) -> ()  [unwired: 4 in, 1 out]
